vi "LV Exp3.vi"() -> ()   [LabVIEW 2009]
uses:
  <vilib>/NXT/Block Support/NXT_InputPort.ctl
  <vilib>/NXT/Dual Mode Library/Waits/Wait_Num(msec).vi
  <vilib>/NXT/Dual Mode Library/Sensors/Sonar_cm.vi
panel:
  in  "stop":bool
  # "HiTechnic Experimenter's Kit\n\n                 Experiment 3 - Six LEDs and Ultrasonic Sensor\nThis program reads the distane with the Ultrasonic sensor\nand outputs the value read to the LEDs connected to B0 - B5.\n\nSee Experimenter's Kit Handbook for the SuperPro for\nmore information or go to www.hitechnic.com. \n\nPort 1 - HiTechnic Prototype Board\nPort 4 - Ultrasonic sensor \n\n(c) HiTechnic 2011"
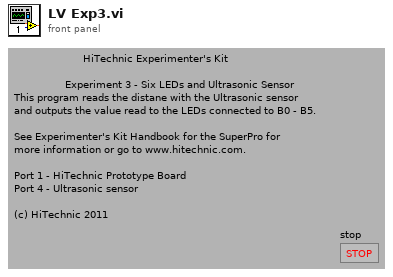
[diagram p1: front panel]
types:
  T1 = typedef "NXT_InputPort.ctl" = u8
  T2 = typedef "LVHSConnector.ctl" = cluster{"error":errorcluster, "address":string, "NXT #":i32, "Show Error":bool, "Connection":u16}
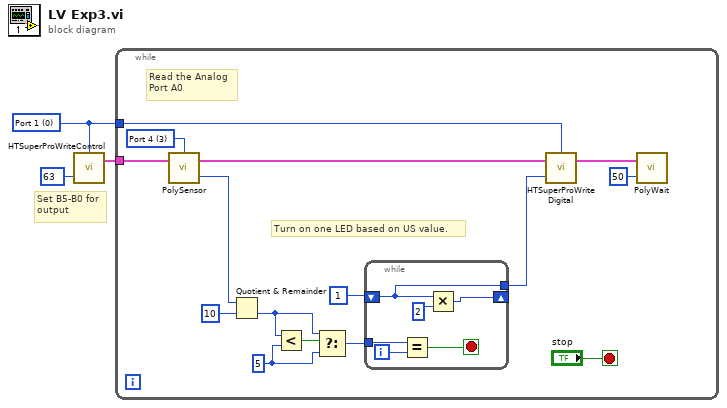
[diagram p0: block diagram]
diagram:
  w1 = T1 0 items=["Port 1", "Port 2", "Port 3", "Port 4"] ("Port")
  # "Set B5-B0 for\noutput"
  n1 = call "HTSuperProWriteControl.vi"("Digital Value"=u8 63, "Port"=w1) -> ("NXT"=w3:T2)  [unwired: 3 in]
  n2 = while {
    tunnel: w1 -> [w18]
    tunnel: w3 -> [w7]
    stop <- "stop" stop-if-true
    w6 = T1 3 items=["Port 1", "Port 2", "Port 3", "Port 4"] ("Port (Port 4)")
    w11 = i16 5 ("y")
    # "Turn on one LED based on US value."
    # "Read the Analog\nPort A0"
    n3 = call-poly <vilib>:"PolySensor.vi"("NXT"=w7, "Port (Port 4)"=w6) -> ("Distance (cm)"=w4:i16, "NXT"=w5:T2)  [unwired: 1 in]
    n4 = Quotient & Remainder(x=w4, y=i16 10) -> (floor(x/y)=w12:i16)  [unwired: 1 out]
    n5 = Less?(x=w12, y=w11) -> (x < y?=w13:bool)
    n6 = Select(t=w12, s=w13, f=w11) -> (s? t:f=w10:i16)
    n7 = while {
      tunnel: w10 -> [w23]
      shift-right: [w20] -> _
      shift-left: u8 1 ("Digital Value") -> [w19]
      tunnel: [w19] -> w14
      i -> [w24]
      stop <- w22 stop-if-true
      n8 = Equal?(x=w23, y=w24) -> (x = y?=w22:bool)
      n9 = Multiply(x=w19, y=u8 2) -> (x*y=w20:u8)
    }
    n10 = call "HTSuperProWriteDigital.vi"("Digital Value"=w14, "NXT"=w5, "Port"=w18) -> ("NXT"=w9:T2)  [unwired: 2 in]
    n11 = call-poly <vilib>:"PolyWait.vi"("Time (100 msec)"=u32 50, "NXT"=w9) -> ()  [unwired: 2 in, 1 out]
  }
